vi "Pre Launch Init.vi"(11 "Input Operator in":refnum<class "ControlPanel.lvclass"> caption="操作者输入") -> (0 "error out":errorcluster caption="错误输出", 3 "Input Operator out":refnum<class "ControlPanel.lvclass"> caption="操作者输出")   [LabVIEW 2014, in "ControlPanel.lvlib" / "ControlPanel.lvclass"]
doc: "(<B>Filename</B>: Actor Framework.lvlib:Actor.lvclass:Pre Launch Init.vi)\n\nDefines behavior that occurs after the Launch Nested Actor method is invoked but before the actor's Actor Core method begins running.\n\nBy default, this method does nothing. A descendant class may override it to define behavior."
uses:
  ControlPanel.lvclass
  ctl/P3AT_Current.ctl
  ControlPanel.lvclass/ControlPanel.ctl
  Global_var/Global_var.vi
  <vilib>/Utility/xml.llb/Read From XML File(array).vi
  <vilib>/Utility/xml.llb/Read From XML File(string).vi
  Wrapper_lib/zsActor/ActorWrapper.lvclass
panel:
  out "XML Elements":string caption="XML元素"
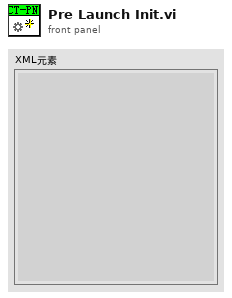
[diagram p1: front panel]
types:
  T1 = typedef "P3AT_Current.ctl" = cluster{"max_vel":dbl, "max_rot":dbl, "now_pose_X":dbl, "now_pose_Y":dbl, "now_pose_Rot_deg":dbl, "Control_Mode":enum32{"Joy", "Map", "Voice", "Input", "Undefined"}}
  T2 = enum16{"OpenSlaveActor", "Idle", "StopSlaveActor"}
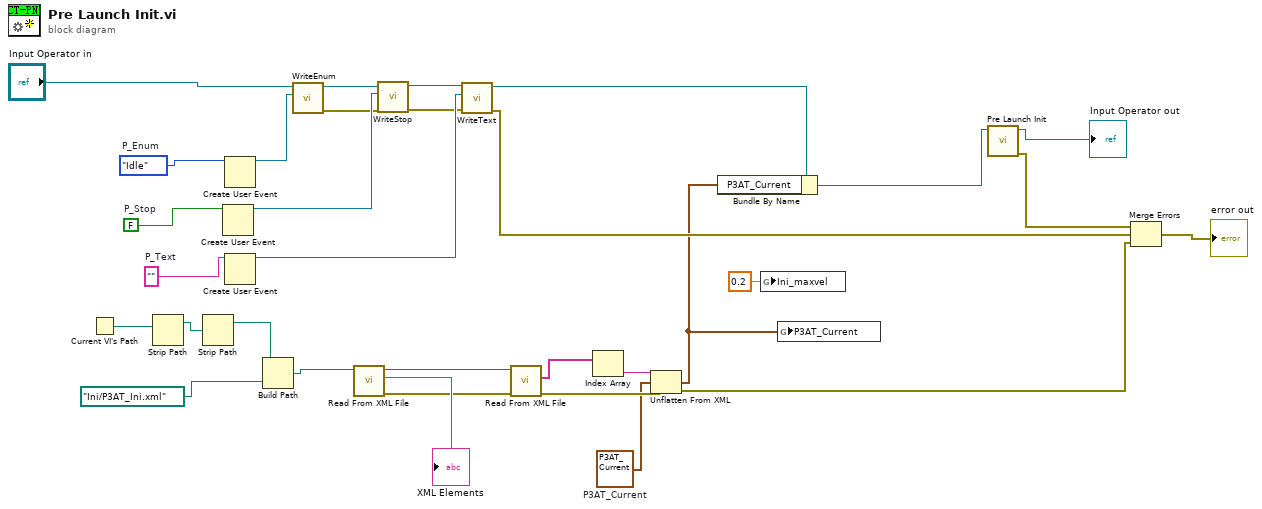
[diagram p0: block diagram]
diagram:
  w2 = T1 {"max_vel"=0.49056603773584906, "max_rot"=0.5094339622641509, "now_pose_X"=0.0, "now_pose_Y"=0.0, "now_pose_Rot_deg"=0.0, "Control_Mode"=enum."Joy"}  # P3AT_Current
  w13 = ""  # P_Text
  w12 = FALSE  # P_Stop
  w11 = T2."Idle"  # P_Enum
  n1 = Current VI's Path() -> (path=w21:path)
  n2 = Strip Path(path=w21) -> (stripped path=w22:path)  [unwired: 1 out]
  n3 = Strip Path(path=w22) -> (stripped path=w23:path)  [unwired: 1 out]
  n4 = Create User Event(user event datatype=w12) -> (user event=w9:refnum<user-event>)  [unwired: 1 in, 1 out]
  n5 = Create User Event(user event datatype=w11) -> (user event=w10:refnum<user-event>)  [unwired: 1 in, 1 out]
  n6 = Create User Event(user event datatype=w13) -> (user event=w8:refnum<user-event>)  [unwired: 1 in, 1 out]
  n7 = Build Path(base path=w23, name or relative path=path "Ini/P3AT_Ini.xml" ("拆分的路径")) -> (appended path=w20:path)
  n8 = call-dynamic "WriteEnum.vi"("Enum"=w10, "zsActor输入"="Input Operator in") -> ("error out"=w7:errorcluster, "zsActor输出"=w16:refnum<class "ControlPanel.lvclass">)  [unwired: 8 in]
  n9 = call-poly <vilib>:"Read From XML File.vi"("XML File Path"=w20) -> ("error out"=w19:errorcluster, "XML Elements"=→"XML Elements":string, "XML File Path(duplicate)"=w28:path)  [unwired: 8 in]
  n10 = call-dynamic "WriteStop.vi"("error in (no error)"=w7, "Stop"=w9, "zsActor输入"=w16) -> ("error out"=w6:errorcluster, "zsActor输出"=w15:refnum<class "ControlPanel.lvclass">)  [unwired: 7 in]
  n11 = call-dynamic "WriteText.vi"("error in (no error)"=w6, "Text"=w8, "zsActor输入"=w15) -> ("error out"=w5:errorcluster, "zsActor输出"=w14:refnum<class "ControlPanel.lvclass">)  [unwired: 7 in]
  n12 = call-poly <vilib>:"Read From XML File.vi"("error in (no error)"=w19, "XML File Path"=w28) -> ("error out"=w18:errorcluster, "XML Elements"=w26:string[])  [unwired: 7 in, 1 out]
  n13 = Index Array(array=w26) -> (element=w25:string)  [unwired: 1 in]
  n14 = Unflatten From XML(xml string=w25, type=w2, error in (no error)=w18) -> (value=w3:T1, error out=w4:errorcluster)
  n15 = Bundle By Name(cluster=w14, "P3AT_Current"=w3) -> (w31:refnum<class "ControlPanel.lvclass">)
  n16 = global write "Global_var.vi" "Ini_maxvel"(0.2 ("Ini_maxvel")) -> ()
  n17 = global write "Global_var.vi" "P3AT_Current"(w3) -> ()
  n18 = call-parent "Pre Launch Init.vi"("Actor in"=w31) -> ("error out"=w30:errorcluster, "Actor out"=→"Input Operator out":refnum<class "ControlPanel.lvclass">)  [unwired: 9 in]
  n19 = Merge Errors(w30, w5, w4) -> (→"error out":errorcluster)
